vi "New JSON Array (JSON Data).vi"(8 "error in (no error)":errorcluster, 10 "JSON Datatypes":refnum<class "JSON Helper.lvclass">[](array[class])) -> (0 "error out":errorcluster, 3 "JSON Array out":refnum<class "JSON Helper.lvclass">)   [LabVIEW 2016, in "JSON Helper.lvclass"]
doc: "Creates a new JSON Array initialized with JSON Boolean objects of the values specified by JSON Datatypes"
uses:
  JSON Helper/JSON Helper.lvclass
  JSON Helper/JSON Helper.lvclass/JSON Helper.ctl
  JSON Types.ctl
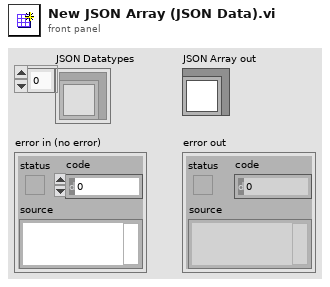
[diagram p1: front panel]
types:
  T1 = typedef "JSON Helper.lvclass/JSON Types.ctl" = enum16{"String", "Numeric", "Boolean", "NULL", "Object", "Array"}
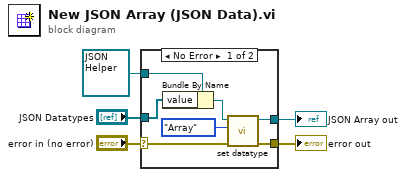
[diagram p0: block diagram]
diagram:
  n1 = case shown="No Error" "error in (no error)" {
    selector: "error in (no error)" -> [w11 w14]
    tunnel: [w9 w14] -> w4
    tunnel: [w7 w13] -> w3
    tunnel: refnum<class "JSON Helper.lvclass"> refnum ("JSON out") -> [w12 w13]
    tunnel: "JSON Datatypes" -> [w10 _]
    frame No Error {
      n2 = Bundle By Name(cluster=w12, "value"=w10) -> (w8:refnum<class "JSON Helper.lvclass">)
      n3 = call "set datatype.vi"("error in (no error)"=w11, "datatype"=JSON_Types."Array", "JSON Helper in"=w8) -> ("error out"=w9:errorcluster, "JSON Helper out"=w7:refnum<class "JSON Helper.lvclass">)  [unwired: 7 in]
    }
    frame Error {
    }
  }
  "error out" <- w4
  "JSON Array out" <- w3
